vi "Research TDMS Image to Word File.vi"() -> ()   [LabVIEW 2021]
uses:
  <vilib>/picture/picture.llb/imagedata.ctl
  Breeeze Utilities/Document/Document.lvclass/Document.ctl
  Breeeze Utilities/Document/Read Word Refs.vi
  Breeeze Utilities/Document/Document.lvclass
  <vilib>/Utility/TDMS File Viewer/NI_TDMS File Viewer.lvlib
  <vilib>/addons/_office/NI_ReportGenerationToolkit.lvlib
  <vilib>/addons/_office/word.llb/Word Find & Replace (str).vi
  <vilib>/Utility/NIReport.llb/Word/NI_Word.lvclass
panel:
  in  "Image information":T1
  out "Img":T2
  out "error out":errorcluster
  in  "Word Templete":path
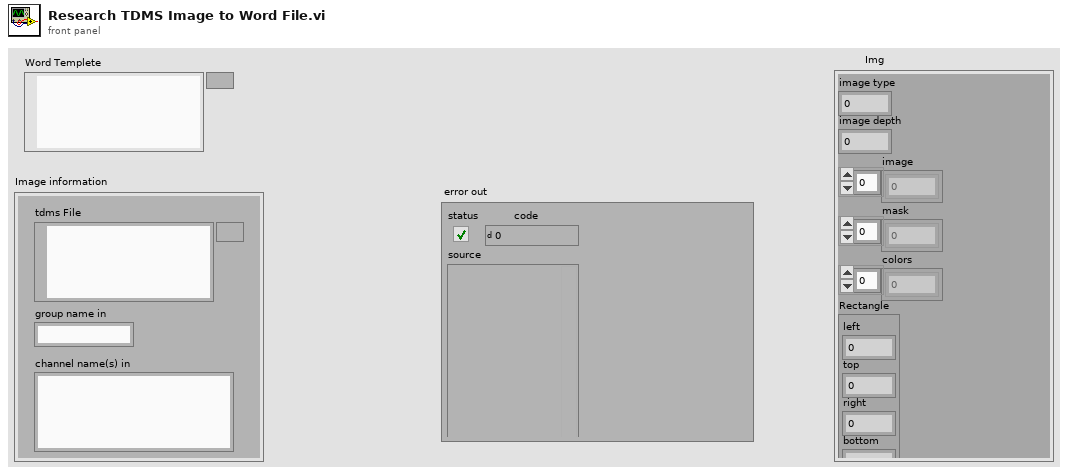
[diagram p1: front panel]
types:
  T1 = cluster{"tdms File":path, "group name in":string, "channel name(s) in":string}
  T2 = typedef "imagedata.ctl" = cluster{"image type":i32, "image depth":i32, "image":u8[], "mask":u8[], "colors":u32[], "Rectangle":cluster{"left":i16, "top":i16, "right":i16, "bottom":i16}}
  T3 = typedef "Breeze Utilities.lvlib/Word Refs Cluster.ctl" = cluster{"Application":refnum<k7>, "Document":refnum<k7>, "Tables":refnum<k7>, "InlineShapes":refnum<k7>, "Documents":refnum<k7>}
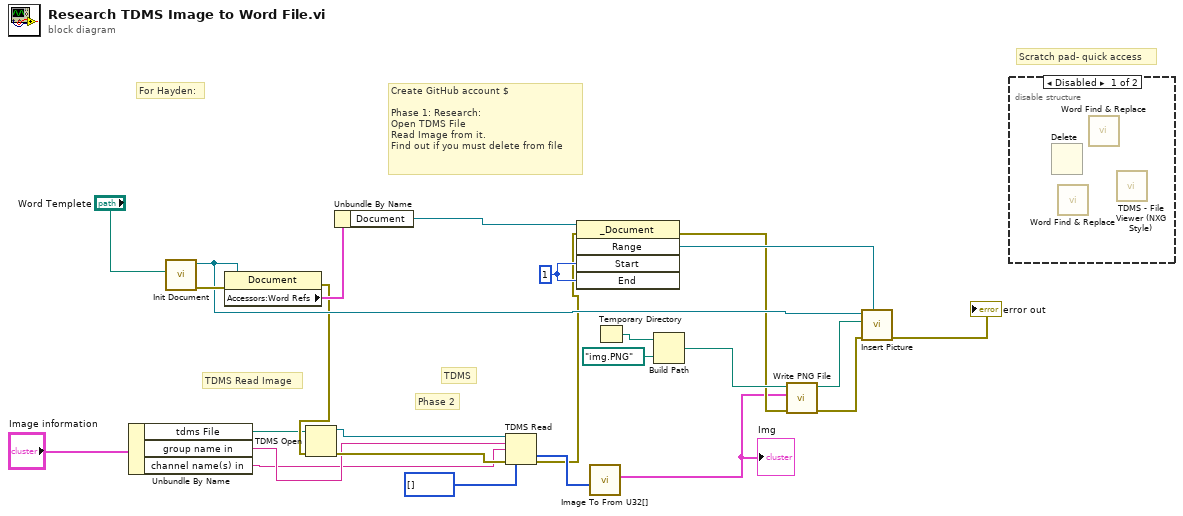
[diagram p0: block diagram]
diagram:
  w19 = 1
  # "Scratch pad- quick access"
  # "TDMS"
  # "Phase 2"
  # "Create GitHub account $\n\nPhase 1: Research:\nOpen TDMS File\nRead Image from it.\nFind out if you must delete from file"
  # "TDMS Read Image"
  # "For Hayden:"
  n1 = Unbundle By Name("Image information") -> ("tdms File"=w3:path, "group name in"=w2:string, "channel name(s) in"=w1:string)
  n2 = call "Init Document.vi"("Template"="Word Templete") -> ("error out"=w23:errorcluster, "Document out"=w15:refnum<class "Document.lvclass">)  [unwired: 9 in]
  n3 = property class="Document"(reference=w15, error in=w23) -> (error out=w10:errorcluster, "Accessors:Word Refs"=w22:T3)  [unwired: 1 out]
  n4 = TDMS Open(8:w10, 11:w3) -> (0:w9:errorcluster, 3:w14:refnum<k34>)  [unwired: 5 in]
  n5 = Unbundle By Name(w22) -> ("Document"=w21:refnum<k7>)
  n6 = TDMS Read(0:w14, 5:w2, 7:w1, 11:w9, 12:u32[] [] ("U32[]")) -> (10:w16:u32[], 15:w8:errorcluster)  [unwired: 3 in, 4 out]
  n7 = invoke class="_Document" method="Range"(reference=w21, error in=w8, "Start"=w19, "End"=w19) -> (error out=w7:errorcluster, "Range"=w20:refnum<k7>)  [unwired: 1 in, 3 out]
  n8 = call "Image To From U32[].vi"("U32[]"=w16) -> ("Img"=w5:T2)  [unwired: 9 in, 1 out]
  "Img" <- w5
  n9 = Temporary Directory() -> (w12:path)
  n10 = Build Path(base path=w12, name or relative path=path "img.PNG") -> (appended path=w25:path)
  n11 = call <vilib>:"Write PNG File.vi"("error in (no error)"=w7, "image data"=w5, "path to PNG file"=w25) -> ("error out"=w6:errorcluster, "path"=w24:path)  [unwired: 7 in]
  n12 = call "Insert Picture.vi"("Range"=w20, "error in (no error)"=w6, "Picture"=w24, "Document in"=w15) -> ("error out"=→"error out":errorcluster)  [unwired: 5 in, 2 out]
  n13 = disable-structure shown="Disabled" {
    frame Disabled {
      n14 = Delete() -> ()  [unwired: 5 in, 3 out]
      n15 = call-poly <vilib>:"Word Find & Replace.vi"() -> ()  [unwired: 13 in, 3 out]
      n16 = call-poly <vilib>:"Word Find & Replace.vi"() -> ()  [unwired: 13 in, 3 out]
      n17 = call <vilib>:"TDMS - File Viewer (NXG Style).vi"() -> ()  [unwired: 10 in, 2 out]
    }
    frame Enabled {
    }
  }
